vi "ADC_Off_Gain_compute(old).vi"(10 "Voltage_Array":dbl[](array[numeric]), 11 "Code":dbl[](array[numeric])) -> (1 "Gain_Error":dbl, 2 "Offset_Error":dbl, 3 "slope":dbl)   [LabVIEW 2019]
uses:
  <vilib>/Analysis/6fits.llb/Curve Fitting Criteria.ctl
  <vilib>/Analysis/NI_AALPro.lvlib
panel:
  out "FS_Error":dbl
  in  "VREF_Measured":dbl=2.5 format="%#_13g"
  out "Meas_Code":dbl
  out "Plot":cluster{dbl[], dbl[]}(graph)
  out "1/x":dbl format="%#_6p"
  out "intercept":dbl
  out "Plots 3":cluster{dbl[], dbl[]}(graph)
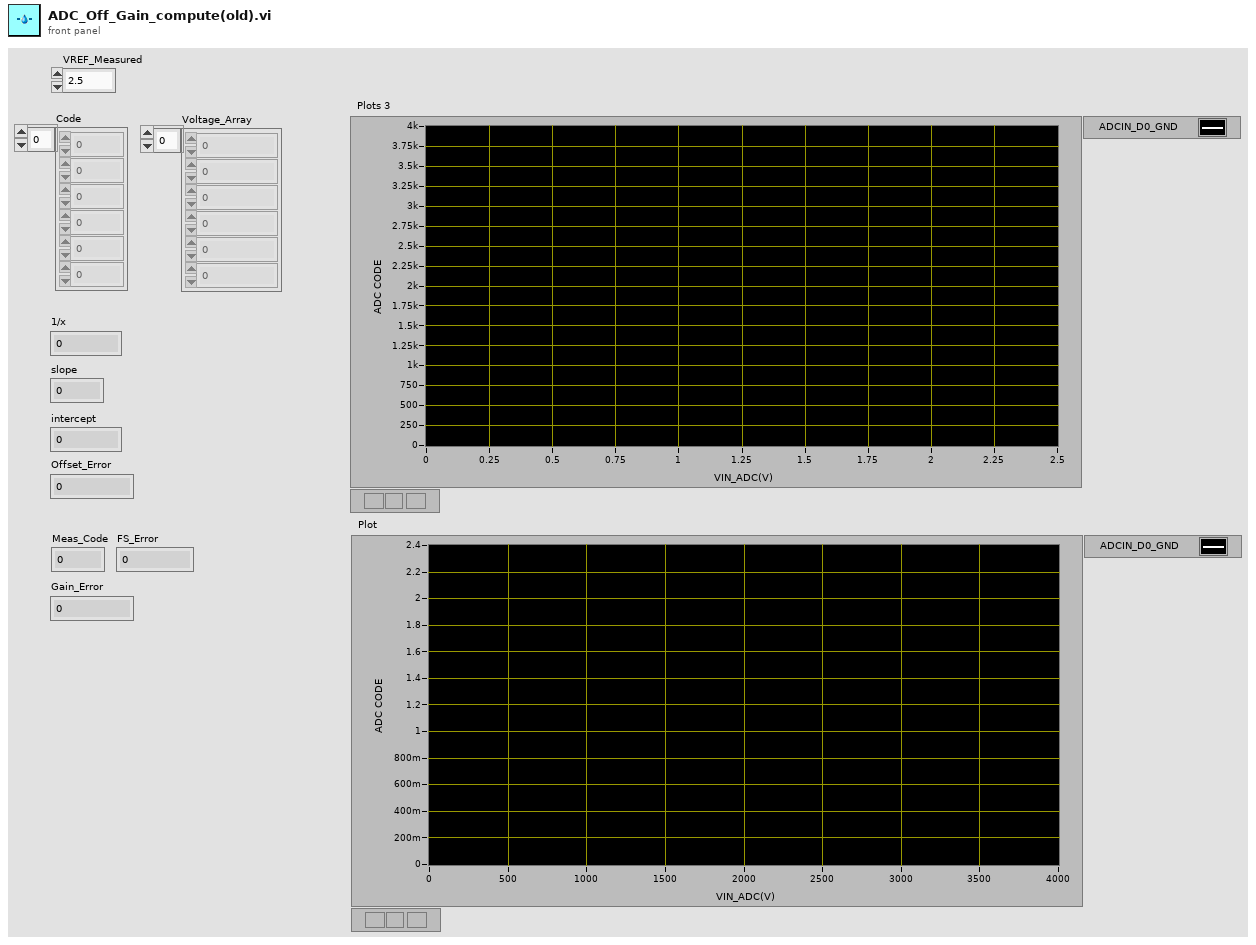
[diagram p1: front panel]
types:
  T1 = typedef "NI_AALPro.lvlib/Curve Fitting Criteria.ctl" = u16
  T2 = cluster{"Voltage_Array":dbl[], "Best Linear Fit":dbl[]}
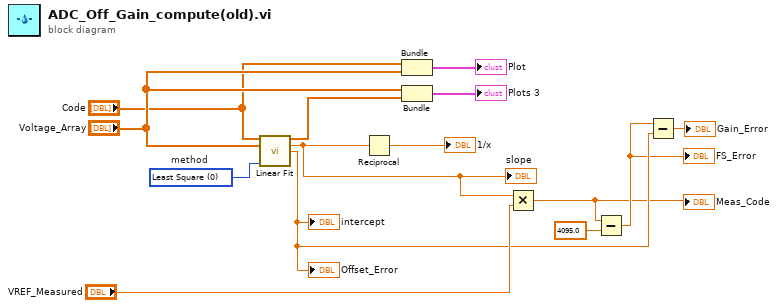
[diagram p0: block diagram]
diagram:
  w14 = T1 0 items=["Least Square", "Least Absolute Residual", "Bisquare"]  # method
  n1 = call <vilib>:"Linear Fit.vi"("Y"="Code", "X"="Voltage_Array", "method"=w14) -> ("Best Linear Fit"=w1:dbl[], "slope"=w7:dbl, "intercept"=w6:dbl)  [unwired: 8 in, 2 out]
  "slope" <- w7
  "intercept" <- w6
  "Offset_Error" <- w6
  n2 = Reciprocal(x=w7) -> (1/x=→"1/x":dbl)
  n3 = Bundle("Code"="Code", "Voltage_Array"="Voltage_Array") -> (→"Plot":cluster{"Code":dbl[], "Voltage_Array":dbl[]})  [unwired: 1 in]
  n4 = Bundle("Voltage_Array"="Voltage_Array", "Best Linear Fit"=w1) -> (→"Plots 3":T2)  [unwired: 1 in]
  n5 = Multiply(x=w7, y="VREF_Measured") -> (x*y=w3:dbl)
  "Meas_Code" <- w3
  n6 = Subtract(x=w3, y=4095.0) -> (x-y=w5:dbl)
  "FS_Error" <- w5
  n7 = Subtract(x=w5, y=w6) -> (x-y=→"Gain_Error":dbl)
